vi "Global 1.vi"() -> ()   [LabVIEW 2014]
panel:
  out "Temperature":dbl
  in  "LED Value":bool
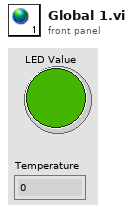
[diagram p1: front panel]
diagram:
